vi "Prepare Build.vi"(8 "error in (no error)":errorcluster, 11 "CD Build Tools in":refnum<class "Project Build Tools.lvclass">) -> (0 "error out":errorcluster, 3 "CD Build Tools out":refnum<class "Project Build Tools.lvclass">)   [LabVIEW 2019, in "Project Build Tools.lvclass"]
uses:
  Project Build Tools.lvclass
  Project Build Tools.lvclass/Project Build Tools.ctl
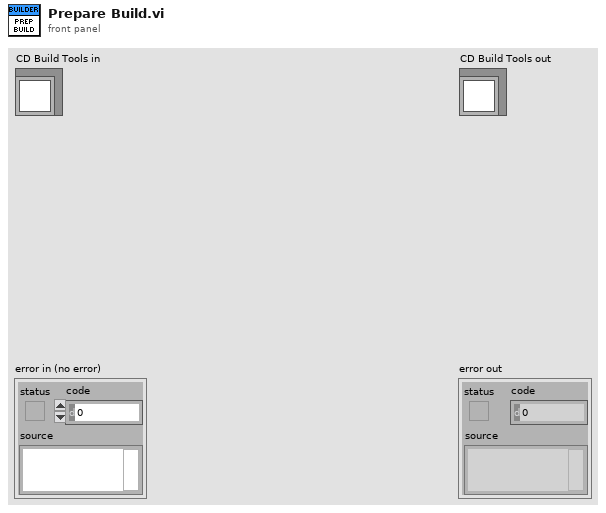
[diagram p1: front panel]
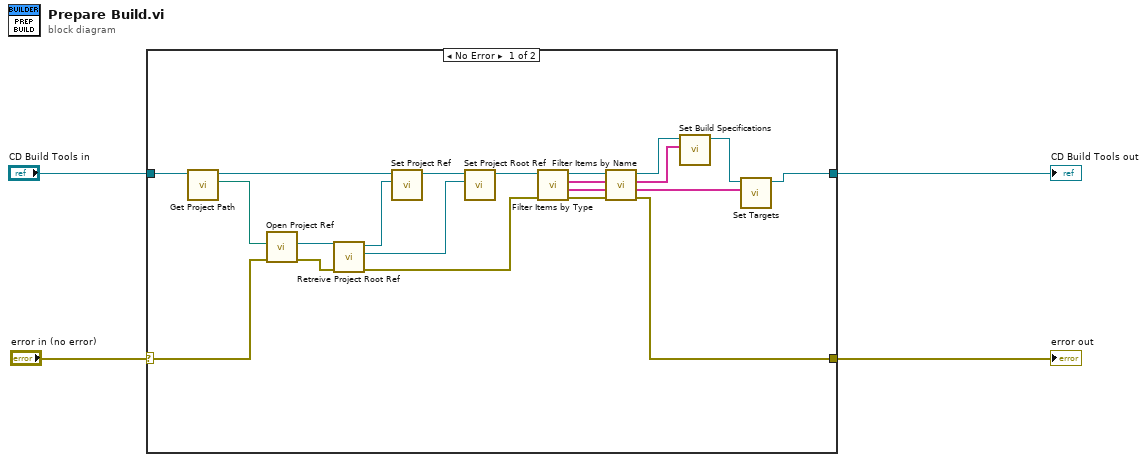
[diagram p0: block diagram]
diagram:
  n1 = case shown="No Error" "error in (no error)" {
    selector: "error in (no error)" -> [w22 w27]
    tunnel: [w11 w27] -> w3
    tunnel: [w6 w26] -> w1
    tunnel: "CD Build Tools in" -> [w25 w26]
    frame No Error {
      n2 = call "Get Project Path.vi"("CD Build Tools in"=w25) -> ("Project Path"=w24:path, "CD Build Tools out"=w20:refnum<class "Project Build Tools.lvclass">)  [unwired: 9 in]
      n3 = call "Open Project Ref.vi"("error in (no error)"=w22, "Project Path"=w24) -> ("error out"=w21:errorcluster, "Project Ref out"=w23:refnum<vi>)  [unwired: 8 in]
      n4 = call "Retreive Project Root Ref.vi"("error in (no error)"=w21, "Project in"=w23) -> ("error out"=w12:errorcluster, "Project Root out"=w18:refnum<vi>, "Project out"=w19:refnum<vi>)  [unwired: 7 in]
      n5 = call "Set Project Ref.vi"("Project Ref"=w19, "CD Build Tools in"=w20) -> ("CD Build Tools out"=w17:refnum<class "Project Build Tools.lvclass">)  [unwired: 9 in]
      n6 = call "Set Project Root Ref.vi"("Project Root Ref"=w18, "CD Build Tools in"=w17) -> ("CD Build Tools out"=w13:refnum<class "Project Build Tools.lvclass">)  [unwired: 9 in]
      n7 = call "Filter Items by Type.vi"("error in (no error)"=w12, "CD Build Tools in"=w13) -> ("error out"=w14:errorcluster, "Target Names"=w8:string[], "Build Specifications out"=w15:string[], "CD Build Tools out"=w16:refnum<class "Project Build Tools.lvclass">)  [unwired: 6 in]
      n8 = call "Filter Items by Name.vi"("error in (no error)"=w14, "Target Names in"=w8, "Build Specifications in"=w15, "CD Build Tools in"=w16) -> ("error out"=w11:errorcluster, "Target Names out"=w5:string[], "Build Specifications out"=w9:string[], "CD Build Tools out"=w10:refnum<class "Project Build Tools.lvclass">)  [unwired: 4 in]
      n9 = call "Set Build Specifications.vi"("Build Specifications"=w9, "CD Build Tools in"=w10) -> ("CD Build Tools out"=w7:refnum<class "Project Build Tools.lvclass">)  [unwired: 9 in]
      n10 = call "Set Targets.vi"("Targets"=w5, "CD Build Tools in"=w7) -> ("CD Build Tools out"=w6:refnum<class "Project Build Tools.lvclass">)  [unwired: 9 in]
    }
    frame Error {
    }
  }
  "error out" <- w3
  "CD Build Tools out" <- w1
